vi "G#Object_GetCommonQueueName.vi"(5 "error in (no error)":errorcluster) -> (14 "queue name":string, 19 "error out":errorcluster)   [LabVIEW 2020, in "G#Object.lvclass"]
doc: "Returns the name of the G# common queue. This is depended on the lib containing the G#Object class. Especially to avoid naming conflict with packed libraries."
uses:
  G#Object.lvclass
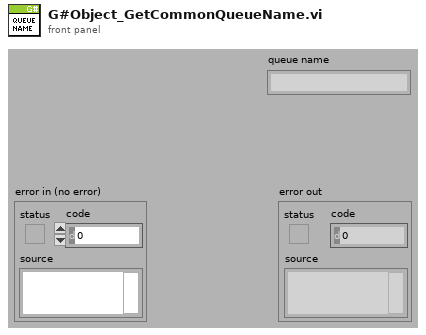
[diagram p1: front panel]
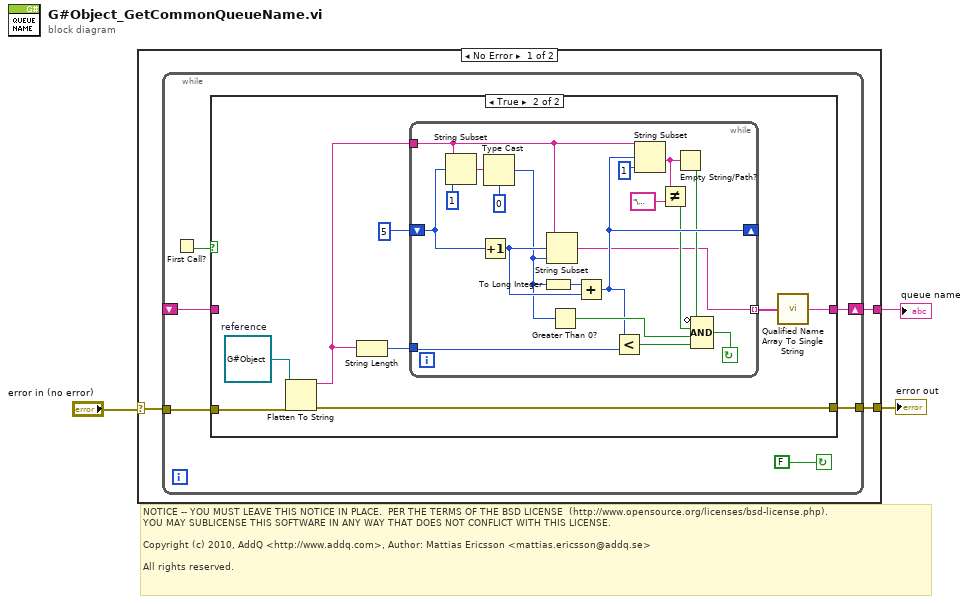
[diagram p0: block diagram]
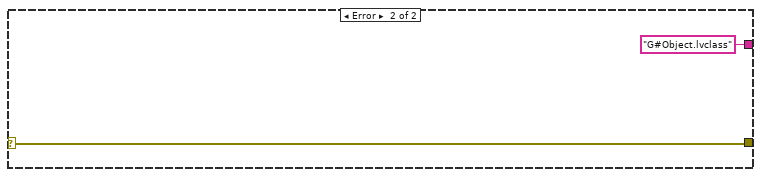
[diagram p3: hidden frame]
diagram:
  # "NOTICE -- YOU MUST LEAVE THIS NOTICE IN PLACE.  PER THE TERMS OF THE BSD LICENSE  (http://www.opensource.org/licenses/bsd-license.php).\nYOU MAY SUBLICENSE THIS SOFTWARE IN ANY WAY THAT DOES NOT CONFLICT WITH THIS LICENSE.\n\nCopyright (c) 2010, AddQ <http://www.addq.com>, Author: Mattias Ericsson <mattias.ericsson@addq.se>\n\nAll rights reserved."
  n1 = case shown="No Error" "error in (no error)" {
    selector: "error in (no error)" -> [w4 w43]
    tunnel: [w6 w43] -> w3
    tunnel: [w5 "G#Object.lvclass" ("Fully Qualified String")] -> w2
    frame No Error {
      n2 = while {
        tunnel: w4 -> [w12]
        tunnel: [w11] -> w6
        shift-right: [w10] -> w5
        shift-left: _ -> [w7]
        stop <- FALSE continue-if-true
        n3 = First Call?() -> (First Call?: T/F=w8:bool)
        n4 = case shown="True" w8 {
          tunnel: w12 -> [w14 w21]
          tunnel: [w14 w20] -> w11
          tunnel: [w13 w15] -> w10
          tunnel: w7 -> [w13 _]
          frame False {
          }
          frame True {
            w22 = refnum<class "G#Object.lvclass"> refnum  # reference
            n5 = Flatten To String(anything=w22, error in (no error)=w21) -> (data string=w16:string, error out=w20:errorcluster)  [unwired: 2 in, 1 out]
            n6 = String Length(string=w16) -> (length=w18:i32)
            n7 = while {
              tunnel: w16 -> [w26]
              shift-right: [w30] -> _
              shift-left: 5 -> [w35]
              tunnel: w18 -> [w37]
              tunnel: [w23] -> w17 mode=indexing
              stop <- w36 continue-if-true
              n8 = String Subset(string=w26, offset (0)=w35, length (rest)=1 ("length (rest)")) -> (substring=w33:string)
              n9 = Increment(x=w35) -> (x+1=w41:i32)
              n10 = Type Cast(type=u8 0 ("default (0 U32)"), x=w33) -> (*(type *) &x=w31:u8)
              n11 = To Long Integer(number=w31) -> (32bit integer=w40:i32)
              n12 = String Subset(string=w26, offset (0)=w41, length (rest)=w31) -> (substring=w23:string)
              n13 = Greater Than 0?(x=w31) -> (x > 0?=w39:bool)
              n14 = Add(x=w40, y=w41) -> (x+y=w30:i32)
              n15 = Less?(x=w30, y=w37) -> (x < y?=w38:bool)
              n16 = String Subset(string=w26, offset (0)=w30, length (rest)=1 ("length (rest)")) -> (substring=w25:string)
              n17 = Not Equal?(x=w25, y="\u0000") -> (x != y?=w27:bool)
              n18 = Empty String/Path?(string/path=w25) -> (empty?=w24:bool)
              n19 = Compound Arithmetic op=AND(invert w24, w27, w39, w38) -> (w36:bool)
            }
            n20 = call <vilib>:"Qualified Name Array To Single String.vi"("Fully Qualified Array"=w17) -> ("Fully Qualified String"=w15:string)
          }
        }
      }
    }
    frame Error {
    }
  }
  "error out" <- w3
  "queue name" <- w2
